vi "Teleop.vi"(10 "Match Info":T1={"Autonomous Elapsed Seconds"=0.0, "TeleOp Elapsed Seconds"=0.0, "Disabled Elapsed Seconds"=0.0, "Visited Autonomous"=FALSE, "Visited TeleOp"=FALSE, "Visited Disabled"=FALSE, "Autonomous Settings"={"Autonomous Style"=enum."Independent", "VI Refnum"=refnum}}, 11 "Call Context":T2) -> ()   [LabVIEW 2014]
doc: "This VI is called for each TeleOp packet received from the DS where the robot is not disabled. It is often used to read from the joysticks and update I/O or to update setpoints for timed control loops. It should complete and return within 20 milliseconds or it may miss DS packets."
uses:
  <vilib>/Rock Robotics/WPI/DriverStation/WPI_DriverStationDerivedRobotMode.ctl
  <vilib>/Rock Robotics/WPI/DriverStation/WPI_DriverStationMatch Info.ctl
  <vilib>/Rock Robotics/WPI/Joystick/WPI_JoystickGetSetRefNum.vi
  <vilib>/Rock Robotics/Network Tables/SD Write Boolean Array.vi
  <vilib>/Rock Robotics/Network Tables/SD Write Numeric Array.vi
  <vilib>/Rock Robotics/Network Tables/SD Read Boolean.vi
  <vilib>/Rock Robotics/Network Tables/SD Read Number.vi
  <vilib>/Rock Robotics/WPI/RobotDrive/WPI_RobotDriveGetSetRefNum.vi
  <vilib>/addons/control/pid/pid.llb/PID Advanced (DBL).vi
  <vilib>/addons/control/pid/NI_PID_pid.lvlib
panel:
  in  "practice bot":bool=TRUE
  in  "stop motors":bool
  in  "set y":dbl format="%#_13g"
  in  "set x":dbl format="%#_13g"
  out "heading":i16
  out "pos y":i16
  out "pos x":i16
  out "distance":fxp<+/-,32,16>[](array[numeric])
  in  "test get data":bool=TRUE
  in  "test drive":bool
  out "Sample Slider 0":dbl(slide) scale=0.0..5.0
  out "Sample Boolean 1":bool
  out "Sample Boolean 0":bool
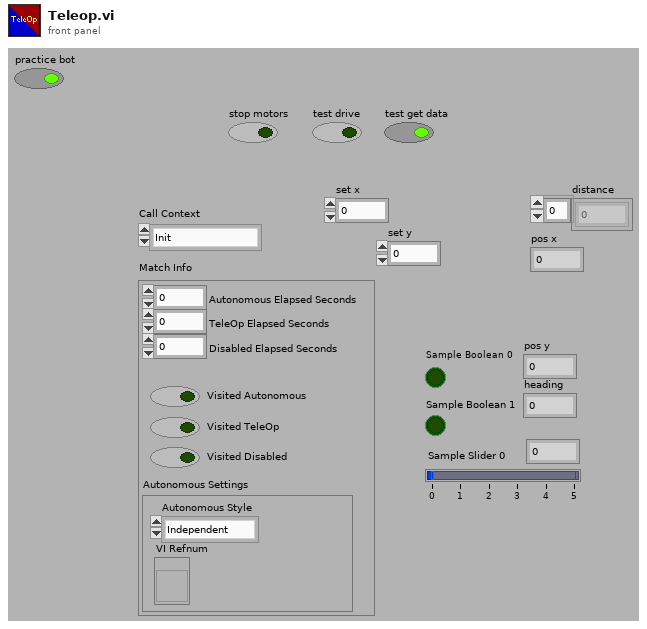
[diagram p1: front panel]
types:
  T1 = typedef "WPI_DriverStationMatch Info.ctl" = cluster{"Autonomous Elapsed Seconds":dbl, "TeleOp Elapsed Seconds":dbl, "Disabled Elapsed Seconds":dbl, "Visited Autonomous":bool, "Visited TeleOp":bool, "Visited Disabled":bool, "Autonomous Settings":cluster{"Autonomous Style":enum16{"Iterative", "Independent"}, "VI Refnum":refnum<vi>}}
  T2 = typedef "WPI_DriverStationDerivedRobotMode.ctl" = enum16{"Init", "Execute", "Stop"}
  T3 = cluster{"proportional gain (Kc)":dbl, "integral time (Ti, min)":dbl, "derivative time (Td, min)":dbl}
  T4 = typedef "WPI_JoystickDevRef.ctl" = cluster{"Device":T5}
  T5 = typedef "WPI_JoystickDeviceEnum.ctl" = enum16{"USB 0", "USB 1", "USB 2", "USB 3", "USB 4", "USB 5"}
  T6 = typedef "WPI_RobotDriveDevRef.ctl" = cluster{"DevStatus":errorcluster, "Motors[]":T7[], "Square Inputs":bool, "Max Output":dbl}
  T7 = typedef "WPI_MotorControlDeviceRef.ctl" = cluster{"DeviceStatus":errorcluster, "Type":T8, "PWM":cluster{"Controller":T9, "PWM Channel":T10, "DeadBand":T11}, "CAN":cluster{"Device Number":u8, "Control Mode":T12, "Semaphore":T13, "Max Vout":dbl, "TalonSRX Control Mode":T14}, "Invert":bool, "TransformRef":T15, "InvTransformRef":T15}
  T8 = typedef "WPI_MotorControlType.ctl" = enum16{"PWM", "CAN", "CANTalonSRX"}
  T9 = typedef "FPGA_TypedefDigitalModule.ctl" = enum16{"Controller 1"}
  T10 = typedef "FPGA_DIOPWMChannel.ctl" = enum8{"PWM 0", "PWM 1", "PWM 2", "PWM 3", "PWM 4", "PWM 5", "PWM 6", "PWM 7", "PWM 8", "PWM 9", "PWM MXP 0", "PWM MXP 1", "PWM MXP 2", "PWM MXP 3", "PWM MXP 4", "PWM MXP 5", "PWM MXP 6", "PWM MXP 7", "PWM MXP 8", "PWM MXP 9", "Invalid"}
  T11 = typedef "WPI_PWMDeadband.ctl" = cluster{"Name":string, "maxPositivePwm":i32, "minPositivePwm":i32, "centerPwm":i32, "maxNegativePwm":i32, "minNegativePwm":i32, "angularRange":u16}
  T12 = typedef "WPI_CANJaguar_ControlMode.ctl" = enum8{"Percent VBus", "Current", "Speed", "Position", "Voltage"}
  T13 = typedef "Semaphore RefNum" = refnum<k1>
  T14 = typedef "WPI_CANTalonSRX_APIControlMode.ctl" = enum8{"Percent VBus", "Speed", "Position", "Slave", "Unchanged / Invalid"}
  T15 = typedef "WPI_PWMTransform_ConPane.ctl" = refnum<vi>
  T16 = cluster{"Axes[0]":dbl, "Axes[1]":dbl, "Axes[2]":dbl, "Axes[3]":dbl, "Axes[4]":dbl, "Axes[5]":dbl, "Axes[6]":dbl, "Axes[7]":dbl, "Axes[8]":dbl}
  T17 = typedef "WPI_EncoderDevRef.ctl" = cluster{"DevStatus":errorcluster, "EncoderIndex":T18, "CounterIndex":T19, "DistancePerCount":dbl, "Decoding Type":T20}
  T18 = typedef "FPGA_EncoderIdx.ctl" = enum8{"Enc 0", "Enc 1", "Enc 2", "Enc 3", "Enc 4", "Enc 5", "Enc 6", "Enc 7", "Invalid"}
  T19 = typedef "FPGA_CounterCtrSystemIndex.ctl" = enum8{"Ctr 0", "Ctr 1", "Ctr 2", "Ctr 3", "Ctr 4", "Ctr 5", "Ctr 6", "Ctr 7", "Invalid"}
  T20 = typedef "WPI_EncoderType.ctl" = enum16{"1x", "2x", "4x"}
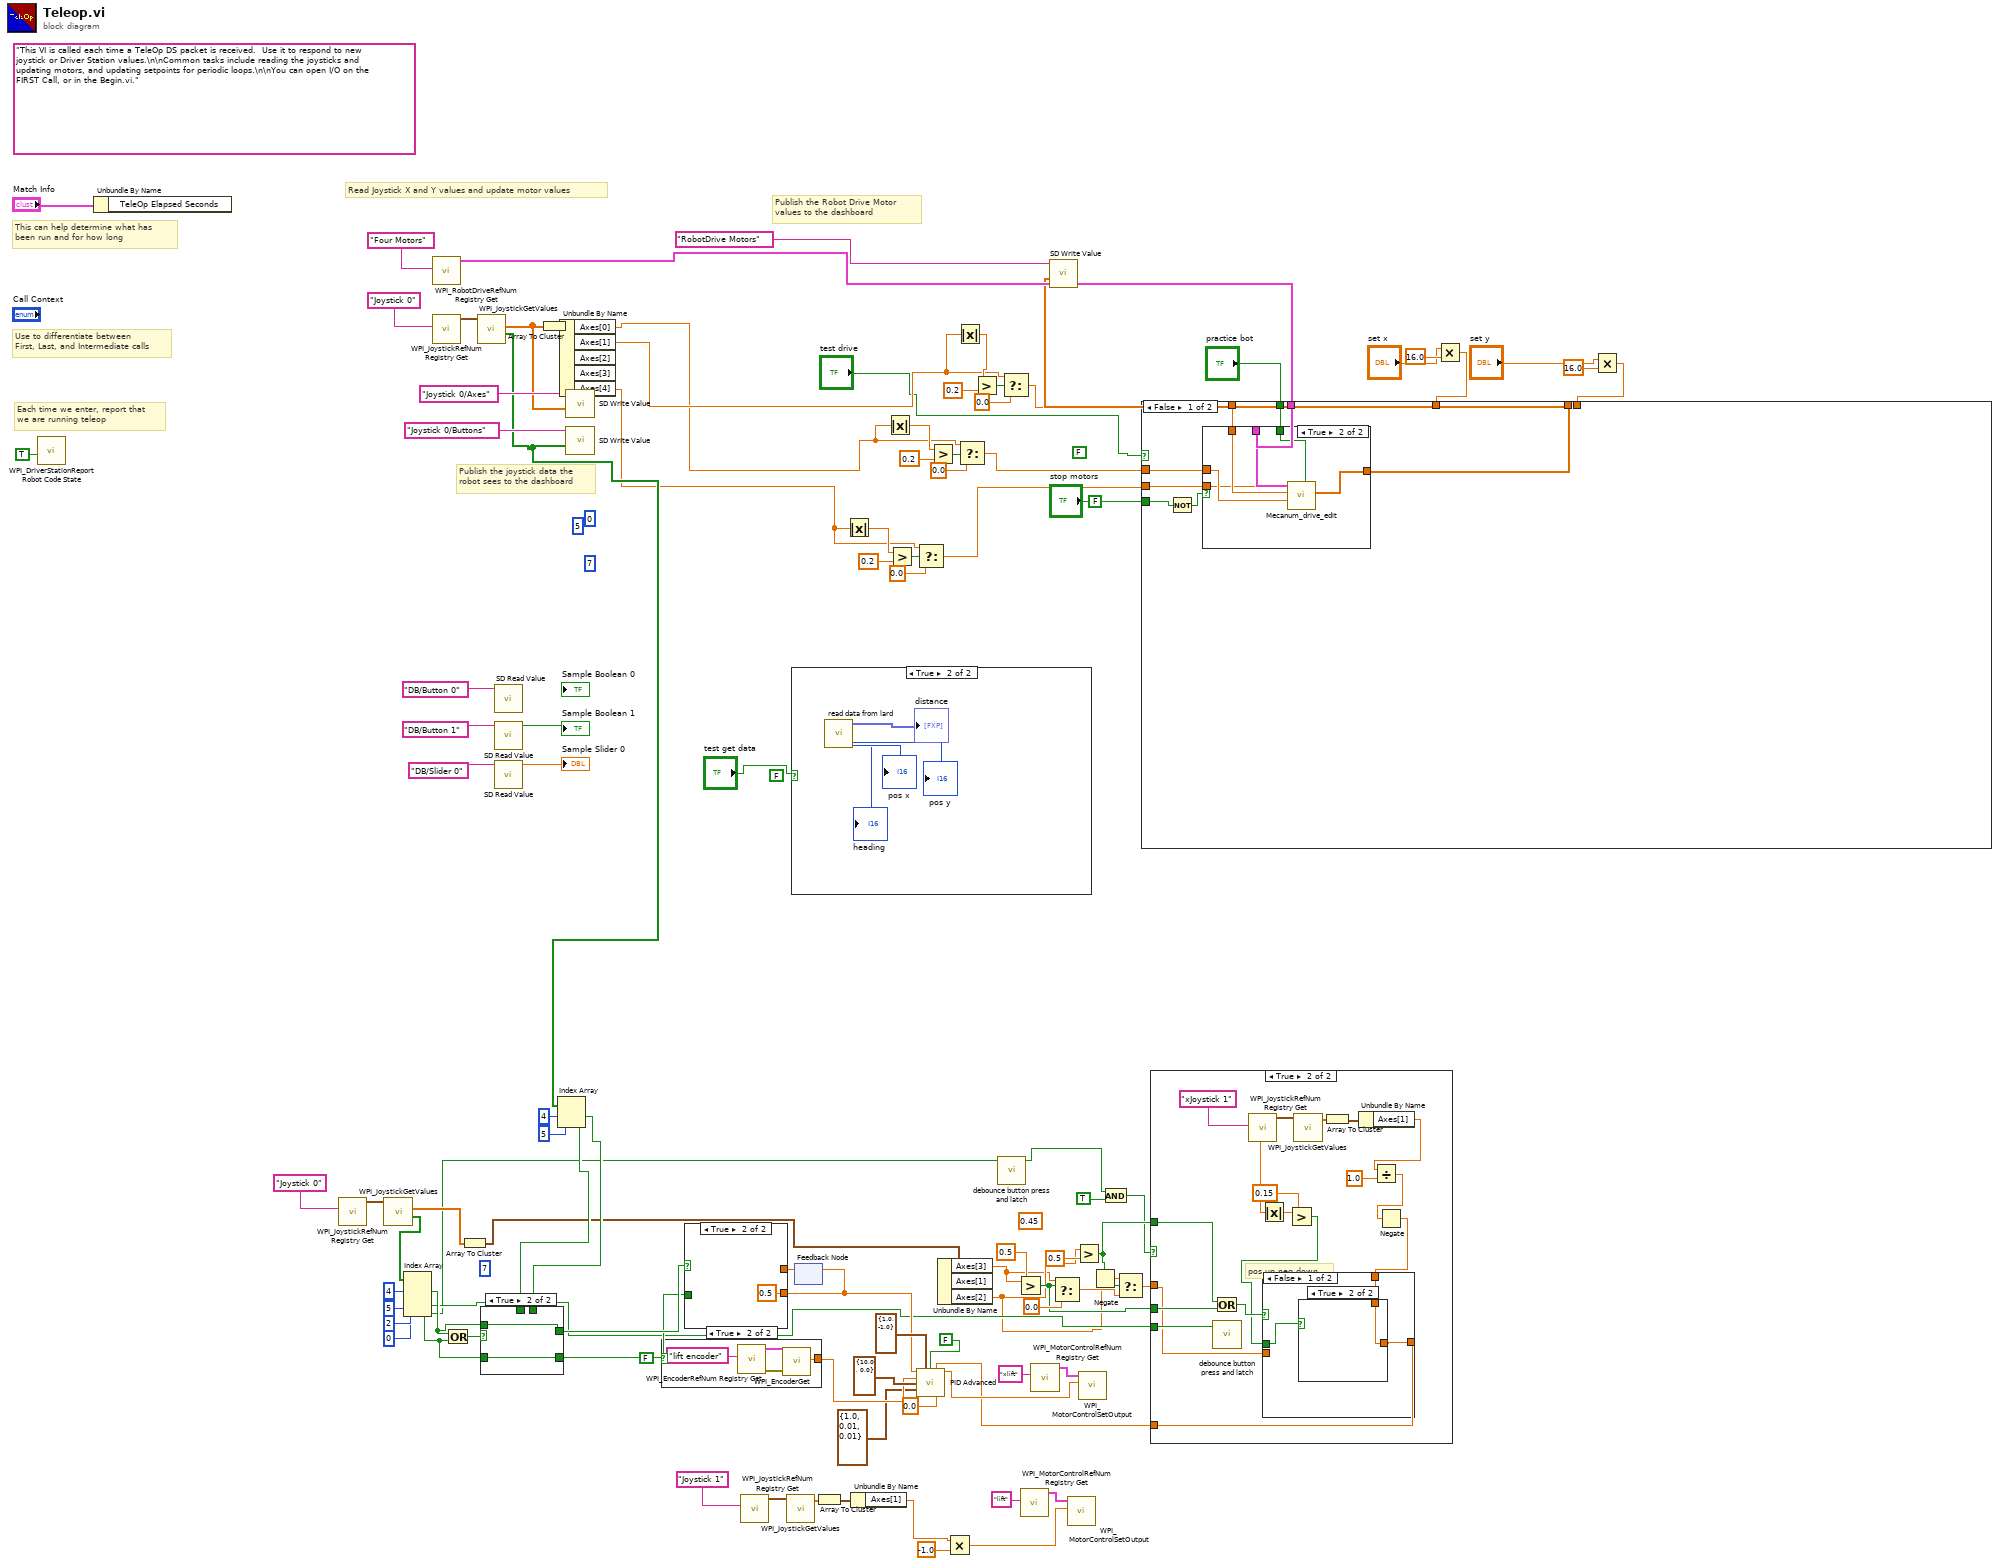
[diagram p0: block diagram]
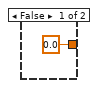
[diagram p4: hidden frame]
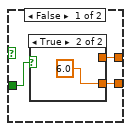
[diagram p7: hidden frame]
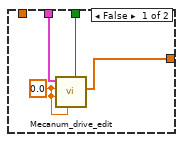
[diagram p10: hidden frame]
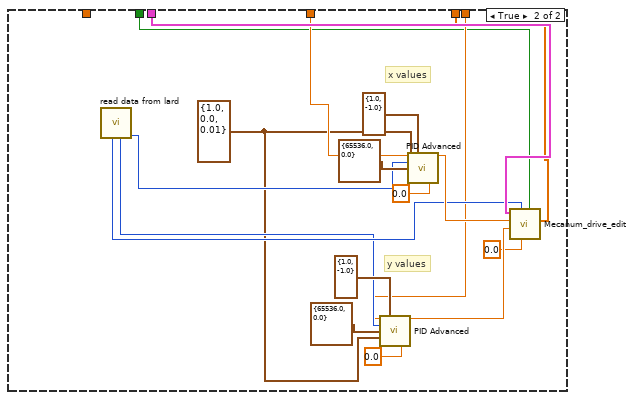
[diagram p11: hidden frame]
diagram:
  (unwired) FALSE
  (unwired) FALSE
  (unwired) FALSE
  (unwired) 0.45 ("t")
  (unwired) 7 ("index")
  (unwired) 7 ("index")
  (unwired) 5 ("index")
  (unwired) 0 ("index")
  (unwired) "This VI is called each time a TeleOp DS packet is received.  Use it to respond to new joystick or Driver Station values.\n\nCommon tasks include reading the joysticks and updating motors, and updating setpoints for periodic loops.\n\nYou can open I/O on the FIRST Call, or in the Begin.vi."
  # "Publish the Robot Drive Motor\nvalues to the dashboard"
  # "Publish the joystick data the\nrobot sees to the dashboard"
  # "Each time we enter, report that\nwe are running teleop"
  # "Use to differentiate between\nFirst, Last, and Intermediate calls"
  # "This can help determine what has\nbeen run and for how long"
  # "Read Joystick X and Y values and update motor values"
  n1 = call <vilib>:"WPI_DriverStationReport Robot Code State.vi"("TeleOp"=TRUE ("Autonomous")) -> ()  [unwired: 10 in, 1 out]
  n2 = Unbundle By Name("Match Info") -> ()  [unwired: 1 out]
  n3 = call <vilib>:"WPI_JoystickRefNum Registry Get.vi"("refnum name"="Joystick 0") -> ("JoystickDevRef"=w65:T4)  [unwired: 1 in, 9 out]
  n4 = call <vilib>:"WPI_JoystickGetValues.vi"("JoystickDevRef"=w65) -> ("Buttons"=w61:bool[], "Axes"=w54:dbl[])  [unwired: 6 in, 3 out]
  n5 = Index Array(array=w61, index #1=4 ("index"), index #2=5 ("index"), index #3=2 ("index"), index #4=0 ("index")) -> (element #1=w59:bool, element #2=w60:bool, element #3=w34:bool, element #4=w24:bool)
  n6 = call <vilib>:"WPI_RobotDriveRefNum Registry Get.vi"("refnum name"="Four Motors") -> ("RobotDriveDevRef"=w86:T6)  [unwired: 1 in, 9 out]
  n7 = call <vilib>:"WPI_JoystickRefNum Registry Get.vi"("refnum name"="Joystick 0") -> ("JoystickDevRef"=w98:T4)  [unwired: 1 in, 9 out]
  n8 = Or(x=w59, y=w60) -> (x .or. y?=w64:bool)
  n9 = Array To Cluster(array=w54) -> (cluster=w53:T16)
  n10 = call <vilib>:"WPI_JoystickGetValues.vi"("JoystickDevRef"=w98) -> ("Buttons"=w67:bool[], "Axes"=w88:dbl[])  [unwired: 6 in, 3 out]
  n11 = call-poly <vilib>:"SD Read Value.vi"("Name"="DB/Button 0" ("refnum name")) -> ()  [unwired: 8 in, 3 out]
  n12 = call-poly <vilib>:"SD Read Value.vi"("Name"="DB/Button 1" ("refnum name")) -> ("Boolean"=→"Sample Boolean 1":bool)  [unwired: 8 in, 2 out]
  n13 = call-poly <vilib>:"SD Read Value.vi"("Name"="DB/Slider 0" ("refnum name")) -> ("Numeric"=→"Sample Slider 0":dbl)  [unwired: 8 in, 2 out]
  n14 = Array To Cluster(array=w88) -> (cluster=w87:T16)
  n15 = Index Array(array=w67, index #1=4 ("index"), index #2=5 ("index")) -> (element #1=w56:bool, element #2=w55:bool)
  n16 = case shown="True" w64 {
    tunnel: [w102 w105] -> w57
    tunnel: w60 -> [_ w105]
    tunnel: [w103 w104] -> w58
    tunnel: w59 -> [_ w104]
    tunnel: w56 -> [w103 _]
    tunnel: w55 -> [w102 _]
    frame False {
    }
    frame True {
    }
  }
  n17 = Unbundle By Name(w87) -> ("Axes[0]"=w35:dbl, "Axes[1]"=w37:dbl, "Axes[4]"=w15:dbl)  [unwired: 2 out]
  n18 = call-poly <vilib>:"SD Write Value.vi"("Numeric Array"=w88, "Name"="Joystick 0/Axes") -> ()  [unwired: 8 in, 2 out]
  n19 = call-poly <vilib>:"SD Write Value.vi"("Boolean Array"=w67, "Name"="Joystick 0/Buttons") -> ()  [unwired: 8 in, 2 out]
  n20 = case shown="True" FALSE {
    tunnel: [_ w107] -> w73
    frame False {
    }
    frame True {
      n21 = call <vilib>:"WPI_EncoderRefNum Registry Get.vi"("refnum name"="lift encoder") -> ("error out"=w109:errorcluster, "EncoderDevRef"=w108:T17)  [unwired: 9 in]
      n22 = call <vilib>:"WPI_EncoderGet.vi"("error in (no error)"=w109, "EncoderDevRef"=w108) -> ("Distance"=w107:dbl)  [unwired: 4 in, 5 out]
    }
  }
  n23 = call <vilib>:"WPI_JoystickRefNum Registry Get.vi"("refnum name"="Joystick 1") -> ("JoystickDevRef"=w9:T4)  [unwired: 1 in, 9 out]
  n24 = call <vilib>:"WPI_JoystickGetValues.vi"("JoystickDevRef"=w9) -> ("Axes"=w8:dbl[])  [unwired: 6 in, 4 out]
  n25 = case shown="True" "test get data" {
    frame False {
    }
    frame True {
      n26 = call "read data from lard.vi"() -> ("pos x"=→"pos x":i16, "distance"=→"distance":fxp<+/-,32,16>[], "pos y"=→"pos y":i16, "heading"=→"heading":i16)  [unwired: 8 in]
    }
  }
  n27 = feedback #1() -> (w68:dbl)  [unwired: 1 in]
  n28 = case shown="True" w58 {
    tunnel: w57 -> [w116 _]
    tunnel: [w115 0.5 ("Output")] -> w69
    tunnel: w68 -> [w114 _]
    frame False {
      n29 = case shown="True" w116 {
        tunnel: [w117 6.0 ("Output")] -> w115
        tunnel: w114 -> [w117 _]
        frame False {
        }
        frame True {
        }
      }
    }
    frame True {
    }
  }
  n30 = feedback-in #1(w69) -> ()
  n31 = Array To Cluster(array=w8) -> (cluster=w7:T16)
  n32 = Absolute Value(x=w15) -> (abs(x)=w16:dbl)
  n33 = Unbundle By Name(w7) -> ("Axes[1]"=w6:dbl)
  n34 = Absolute Value(x=w35) -> (abs(x)=w36:dbl)
  n35 = Greater?(x=w16, y=0.2) -> (0:w19:bool)
  n36 = Select(t=w15, s=w19, f=0.0) -> (s? t:f=w14:dbl)
  n37 = Greater?(x=w36, y=0.2) -> (0:w43:bool)
  n38 = Unbundle By Name(w53) -> ("Axes[3]"=w1:dbl, "Axes[2]"=w2:dbl)  [unwired: 1 out]
  n39 = Multiply(x=w6, y=-1.0) -> (x*y=w5:dbl)
  n40 = Absolute Value(x=w37) -> (abs(x)=w38:dbl)
  n41 = Select(t=w35, s=w43, f=0.0) -> (s? t:f=w41:dbl)
  n42 = Greater?(x=w38, y=0.2) -> (0:w46:bool)
  n43 = call "debounce button press and latch.vi"("Boolean"=w24) -> ("Boolean 2"=w27:bool)  [unwired: 10 in]
  n44 = Select(t=w37, s=w46, f=0.0) -> (s? t:f=w45:dbl)
  n45 = Greater?(x=w1, y=0.5) -> (0:w33:bool)
  n46 = call <vilib>:"WPI_MotorControlRefNum Registry Get.vi"("refnum name"="lift") -> ("MotorControlDevRef"=w11:T7)  [unwired: 9 in, 1 out]
  n47 = call <vilib>:"WPI_MotorControlRefNum Registry Get.vi"("refnum name"="xlift") -> ("MotorControlDevRef"=w70:T7)  [unwired: 9 in, 1 out]
  n48 = Select(t=w1, s=w33, f=0.0) -> (s? t:f=w31:dbl)
  n49 = call <vilib>:"WPI_MotorControlSetOutput.vi"("Output"=w5, "MotorControlDevRef"=w11) -> ()  [unwired: 7 in, 3 out]
  n50 = Greater?(x=w2, y=0.5) -> (0:w30:bool)
  n51 = Negate(x=w2) -> (-x=w3:dbl)
  n52 = And(x=w27, y=TRUE) -> (x .and. y?=w28:bool)
  n53 = Select(t=w3, s=w30, f=w31) -> (s? t:f=w29:dbl)
  n54 = case shown="True" w28 {
    tunnel: w34 -> [_ w137]
    tunnel: w33 -> [_ w131]
    tunnel: [w120 w129] -> w32
    tunnel: w30 -> [_ w125]
    tunnel: w29 -> [w120 w124]
    frame False {
    }
    frame True {
      # "pos up neg down"
      n55 = Or(x=w125, y=w131) -> (x .or. y?=w132:bool)
      n56 = call "debounce button press and latch.vi"("Boolean"=w137) -> ()  [unwired: 10 in, 1 out]
      n57 = call <vilib>:"WPI_JoystickRefNum Registry Get.vi"("refnum name"="xJoystick 1") -> ("JoystickDevRef"=w135:T4)  [unwired: 1 in, 9 out]
      n58 = call <vilib>:"WPI_JoystickGetValues.vi"("JoystickDevRef"=w135) -> ("Axes"=w134:dbl[])  [unwired: 6 in, 4 out]
      n59 = Array To Cluster(array=w134) -> (cluster=w133:T16)
      n60 = Unbundle By Name(w133) -> ("Axes[1]"=w123:dbl)
      n61 = Absolute Value(x=w123) -> (abs(x)=w128:dbl)
      n62 = Greater?(x=w128, y=0.15) -> (0:w126:bool)
      n63 = Divide(x=w123, y=1.0) -> (x/y=w121:dbl)
      n64 = Negate(x=w121) -> (-x=w130:dbl)
      n65 = case shown="False" w132 {
        tunnel: w126 -> [w140 _]
        tunnel: [w139 w143] -> w129
        tunnel: w124 -> [_ w143]
        tunnel: w130 -> [w138 _]
        frame False {
          n66 = case shown="True" w140 {
            tunnel: [0.0 w142] -> w139
            tunnel: w138 -> [_ w142]
            frame False {
            }
            frame True {
            }
          }
        }
        frame True {
        }
      }
    }
  }
  n67 = call-poly <vilib>:"PID Advanced.vi"("setpoint"=w69, "output range"=cluster{"output high":dbl, "output low":dbl} {"output high"=1.0, "output low"=-1.0}, "auto? (T)"=FALSE, "manual control"=w32, "process variable"=w73, "setpoint range"=cluster{"setpoint high":dbl, "setpoint low":dbl} {"setpoint high"=10.0, "setpoint low"=0.0}, "PID gains"=T3 {"proportional gain (Kc)"=1.0, "integral time (Ti, min)"=0.01, "derivative time (Td, min)"=0.01}, "linearity"=0.0) -> ("output"=w47:dbl)  [unwired: 6 in, 1 out]
  n68 = call <vilib>:"WPI_MotorControlSetOutput.vi"("Output"=w47, "MotorControlDevRef"=w70) -> ()  [unwired: 7 in, 3 out]
  n69 = Multiply(x="set x", y=16.0) -> (x*y=w80:dbl)
  n70 = Multiply(x="set y", y=16.0) -> (x*y=w79:dbl)
  n71 = case shown="False" "test drive" {
    tunnel: w86 -> [w151 w170]
    tunnel: w45 -> [w150 _]
    tunnel: w41 -> [w149 _]
    tunnel: [w148 w163] -> w85
    tunnel: w14 -> [w147 _]
    tunnel: w80 -> [_ w166]
    tunnel: w79 -> [_ w165]
    tunnel: "stop motors" -> [w145 _]
    tunnel: "practice bot" -> [w144 w162]
    frame False {
      n72 = Not(x=w145) -> (.not. x?=w146:bool)
      n73 = case shown="True" w146 {
        tunnel: w151 -> [w155 w161]
        tunnel: w150 -> [_ w160]
        tunnel: w149 -> [_ w159]
        tunnel: [w153 w158] -> w148
        tunnel: w147 -> [_ w157]
        tunnel: w144 -> [w152 w156]
        frame False {
          w154 = 0.0 ("X")
          n74 = call "Mecanum_drive_edit.vi"("practice bot"=w152, "Rotation"=w154, "Y"=w154, "X"=w154, "RobotDriveDevRef"=w155) -> ("Motor Values"=w153:dbl[])  [unwired: 4 in, 2 out]
        }
        frame True {
          n75 = call "Mecanum_drive_edit.vi"("practice bot"=w156, "Rotation"=w157, "Y"=w159, "X"=w160, "RobotDriveDevRef"=w161) -> ("Motor Values"=w158:dbl[])  [unwired: 4 in, 2 out]
        }
      }
    }
    frame True {
      w164 = T3 {"proportional gain (Kc)"=1.0, "integral time (Ti, min)"=0.0, "derivative time (Td, min)"=0.01} ("PID gains")
      # "y values"
      # "x values"
      n76 = call "read data from lard.vi"() -> ("pos x"=w168:i16, "pos y"=w167:i16, "heading"=w169:i16)  [unwired: 8 in, 1 out]
      n77 = call-poly <vilib>:"PID Advanced.vi"("setpoint"=w165, "output range"=cluster{"output high":dbl, "output low":dbl} {"output high"=1.0, "output low"=-1.0}, "process variable"=w167, "setpoint range"=cluster{"setpoint high":dbl, "setpoint low":dbl} {"setpoint high"=65536.0, "setpoint low"=0.0}, "PID gains"=w164, "linearity"=0.0) -> ("output"=w172:dbl)  [unwired: 8 in, 1 out]
      n78 = call-poly <vilib>:"PID Advanced.vi"("setpoint"=w166, "output range"=cluster{"output high":dbl, "output low":dbl} {"output high"=1.0, "output low"=-1.0}, "process variable"=w168, "setpoint range"=cluster{"setpoint high":dbl, "setpoint low":dbl} {"setpoint high"=65536.0, "setpoint low"=0.0}, "PID gains"=w164, "linearity"=0.0) -> ("output"=w173:dbl)  [unwired: 8 in, 1 out]
      n79 = call "Mecanum_drive_edit.vi"("practice bot"=w162, "Rotation"=0.0, "Gyro Angle"=w169, "Y"=w172, "X"=w173, "RobotDriveDevRef"=w170) -> ("Motor Values"=w163:dbl[])  [unwired: 3 in, 2 out]
    }
  }
  n80 = call-poly <vilib>:"SD Write Value.vi"("Numeric Array"=w85, "Name"="RobotDrive Motors") -> ()  [unwired: 8 in, 2 out]
